vi "MNIST_Read_Dataset(as3D_refs).vi"(7 "MNIST Dataset Path":path=path "D:/DNN/data/DataSets/MNIST/train-images.idx3-ubyte", 8 "error in":errorcluster, 10 "Validation_Size":sgl=0.1) -> (0 "error out":errorcluster, 3 "Data(3D)_Refs":T1={"Train"={"Inputs Ref."=variant(refnum<data-value> refnum), "Outputs Ref."=refnum, "Dataset_Size"=0, "Dims_In"={"C"=0, "H"=0, "W"=0}, "Dims_Out"=0, "Labels"=[], "File Paths"=[]}, "Validation"={"Inputs Ref."=variant(refnum<data-value> refnum), "Outputs Ref."=refnum, "Dataset_Size"=0, "Dims_In"={"C"=0, "H"=0, "W"=0}, "Dims_Out"=0, "Labels"=[], "File Paths"=[]}, "Test"={"Inputs Ref."=variant(refnum<data-value> refnum), "Outputs Ref."=refnum, "Dataset_Size"=0, "Dims_In"={"C"=0, "H"=0, "W"=0}, "Dims_Out"=0, "Labels"=[], "File Paths"=[]}})   [LabVIEW 2024]
doc: "References to the dataset (Training, Validation and Testing)"
uses:
  <vilib>/Ngene/Deep Learning Toolkit/Toolkit/NN_Data/API/DataSet/DataSet_Types/NN_DataSets_All(In3D_Out1D).ctl
  <vilib>/Ngene/Deep Learning Toolkit/Toolkit/NN_Data/API/DataSet/DataSet_Types/NN_DataSet(In3D_Out1D).ctl
  <vilib>/Ngene/Deep Learning Toolkit/Toolkit/NN_Data/Controls/DataRef_Types/2D/NN_Data_ref(2D_SGL).ctl
  <vilib>/Ngene/Deep Learning Toolkit/Toolkit/NN_Data/API/NN_Dims(C,H,W).ctl
  <vilib>/Ngene/Deep Learning Toolkit/Toolkit/NN_Data/subVIs/Dataset_Split/NN_DataSet_Split(In3D_Out1D).vi
  <vilib>/Ngene/Deep Learning Toolkit/Toolkit/Deep_Learning_Toolkit_by_Ngene.lvlib
panel:
  # "Instructions:\n1. Download MNIST dataset from http://yann.lecun.com/exdb/mnist/  (4 files with .gz extension)\n2. Extract all 4 files in one folder\n3.  Provide corresponding path to 4 path controls below"
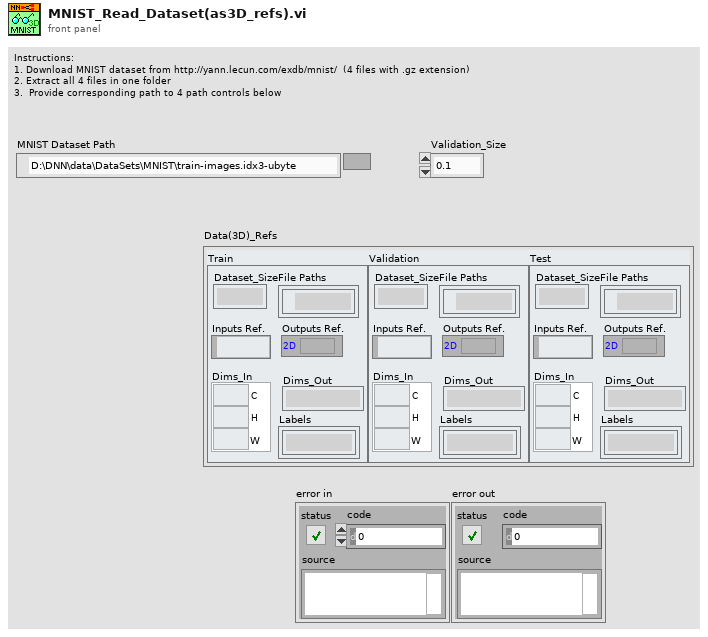
[diagram p1: front panel]
types:
  T1 = typedef "Deep_Learning_Toolkit_by_Ngene.lvlib/NN_DataSets_All(In3D_Out1D).ctl" = cluster{"Train":T2, "Validation":T2, "Test":T2}
  T2 = typedef "Deep_Learning_Toolkit_by_Ngene.lvlib/NN_DataSet(In3D_Out1D).ctl" = cluster{"Inputs Ref.":variant, "Outputs Ref.":T3, "Dataset_Size":i32, "Dims_In":T4, "Dims_Out":i32, "Labels":string[], "File Paths":path[]}
  T3 = typedef "Deep_Learning_Toolkit_by_Ngene.lvlib/NN_Data_ref(2D_SGL).ctl" = refnum<data-value>
  T4 = typedef "Deep_Learning_Toolkit_by_Ngene.lvlib/NN_Dims(C,H,W).ctl" = cluster{"C":i32, "H":i32, "W":i32}
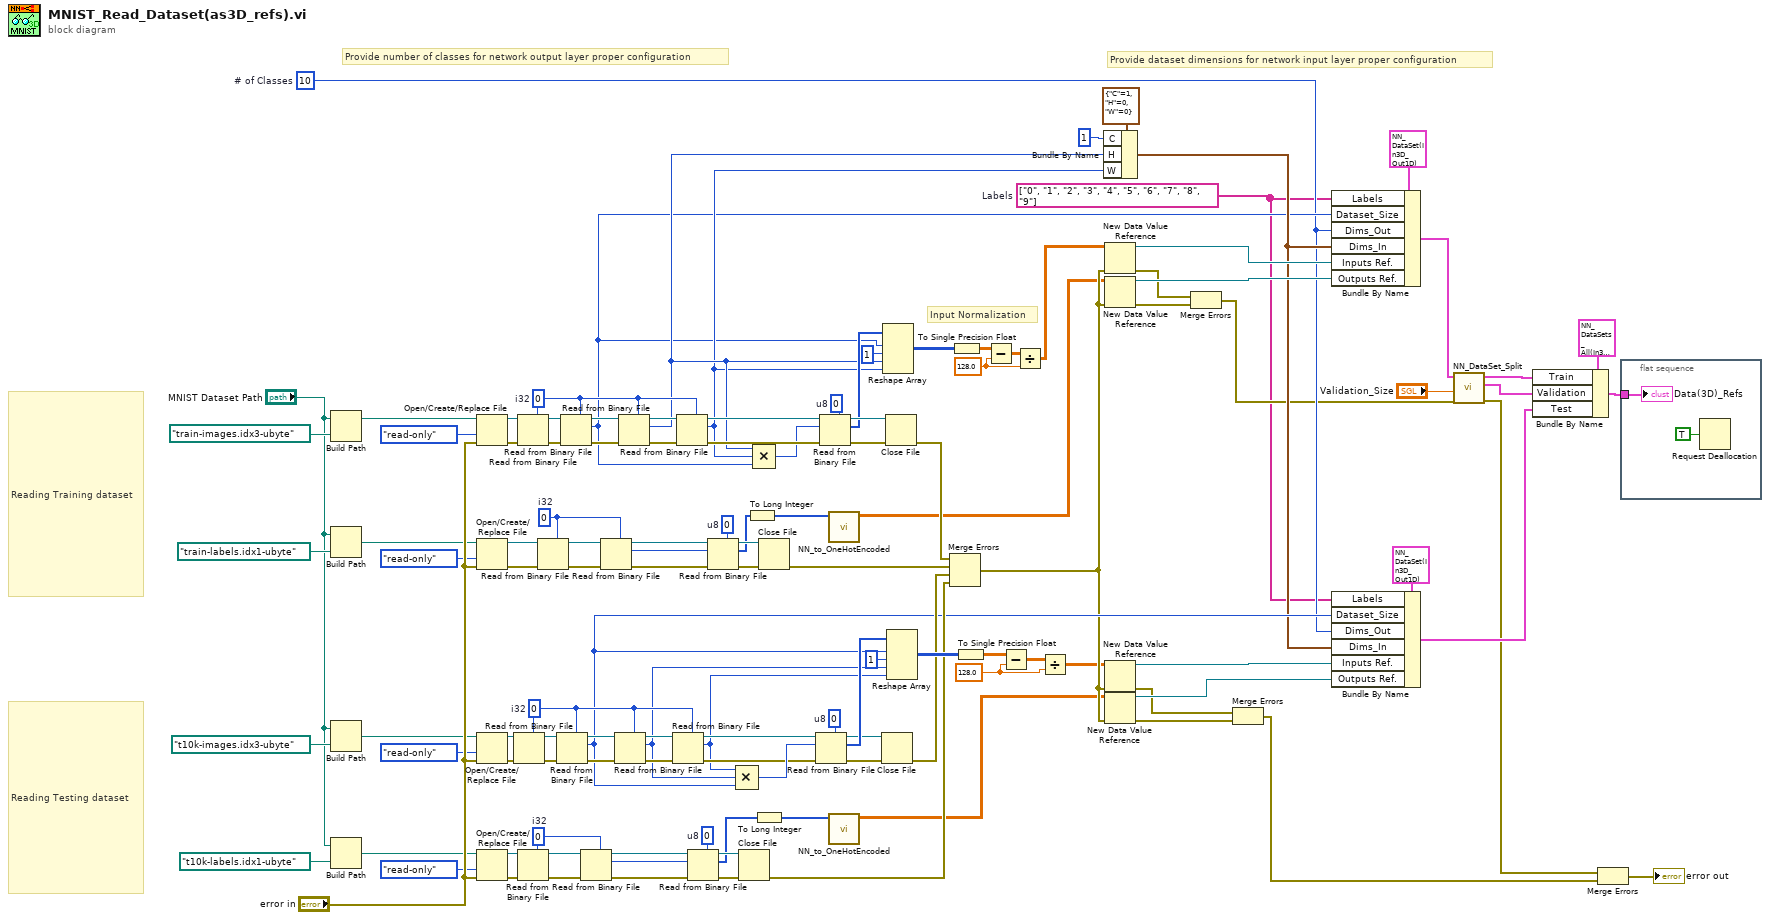
[diagram p0: block diagram]
diagram:
  w5 = string[] ["0", "1", "2", "3", "4", "5", "6", "7", "8", "9"]  # Labels
  w22 = sgl 128.0 ("y")
  w24 = sgl 128.0 ("y")
  w12 = 10  # # of Classes
  w94 = u8 0  # u8
  w93 = u8 0  # u8
  w85 = 0  # i32
  w74 = 0  # i32
  w98 = u8 0  # u8
  w99 = u8 0  # u8
  w107 = 0  # i32
  w118 = 0  # i32
  # "Provide dataset dimensions for network input layer proper configuration"
  # "Provide number of classes for network output layer proper configuration"
  # "Reading Testing dataset"
  # "Reading Training dataset"
  # "Input Normalization"
  n1 = Build Path(base path="MNIST Dataset Path", name or relative path=path "train-images.idx3-ubyte" ("Train_Label_Path")) -> (appended path=w21:path)
  n2 = Build Path(base path="MNIST Dataset Path", name or relative path=path "train-labels.idx1-ubyte" ("Train_Label_Path")) -> (appended path=w20:path)
  n3 = Build Path(base path="MNIST Dataset Path", name or relative path=path "t10k-images.idx3-ubyte" ("Test_Image_Path")) -> (appended path=w17:path)
  n4 = Build Path(base path="MNIST Dataset Path", name or relative path=path "t10k-labels.idx1-ubyte" ("Test_Label_Path")) -> (appended path=w14:path)
  n5 = Open/Create/Replace File(file path (use dialog)=w21, error in="error in", access (0:read/write)=enum16{"read/write", "read-only", "write-only"}."read-only") -> (refnum out=w122:refnum<file>, error out=w116:errorcluster)  [unwired: 3 in, 1 out]
  n6 = Open/Create/Replace File(file path (use dialog)=w20, error in="error in", access (0:read/write)=enum16{"read/write", "read-only", "write-only"}."read-only") -> (refnum out=w105:refnum<file>, error out=w108:errorcluster)  [unwired: 3 in, 1 out]
  n7 = Open/Create/Replace File(file path (use dialog)=w17, error in="error in", access (0:read/write)=enum16{"read/write", "read-only", "write-only"}."read-only") -> (refnum out=w70:refnum<file>, error out=w76:errorcluster)  [unwired: 3 in, 1 out]
  n8 = Open/Create/Replace File(file path (use dialog)=w14, error in="error in", access (0:read/write)=enum16{"read/write", "read-only", "write-only"}."read-only") -> (refnum out=w87:refnum<file>, error out=w84:errorcluster)  [unwired: 3 in, 1 out]
  n9 = Read from Binary File(5:w74, 8:w76, 11:w70) -> (0:w77:errorcluster, 3:w71:refnum<file>)  [unwired: 3 in, 2 out]
  n10 = Read from Binary File(5:w118, 8:w116, 11:w122) -> (0:w115:errorcluster, 3:w121:refnum<file>)  [unwired: 3 in, 2 out]
  n11 = Read from Binary File(5:w85, 8:w84, 11:w87) -> (0:w83:errorcluster, 3:w86:refnum<file>)  [unwired: 3 in, 2 out]
  n12 = Read from Binary File(5:w107, 8:w108, 11:w105) -> (0:w109:errorcluster, 3:w106:refnum<file>)  [unwired: 3 in, 2 out]
  n13 = Read from Binary File(5:w74, 8:w77, 11:w71) -> (0:w78:errorcluster, 2:w49:i32, 3:w73:refnum<file>)  [unwired: 3 in, 1 out]
  n14 = Read from Binary File(5:w118, 8:w115, 11:w121) -> (0:w114:errorcluster, 2:w26:i32, 3:w119:refnum<file>)  [unwired: 3 in, 1 out]
  n15 = Read from Binary File(5:w85, 8:w83, 11:w86) -> (0:w89:errorcluster, 2:w43:i32, 3:w88:refnum<file>)  [unwired: 3 in, 1 out]
  n16 = Read from Binary File(5:w107, 8:w109, 11:w106) -> (0:w103:errorcluster, 2:w44:i32, 3:w104:refnum<file>)  [unwired: 3 in, 1 out]
  n17 = Read from Binary File(5:w74, 8:w78, 11:w73) -> (0:w79:errorcluster, 2:w35:i32, 3:w72:refnum<file>)  [unwired: 3 in, 1 out]
  n18 = Read from Binary File(5:w118, 8:w114, 11:w119) -> (0:w113:errorcluster, 2:w30:i32, 3:w120:refnum<file>)  [unwired: 3 in, 1 out]
  n19 = Read from Binary File(5:w74, 8:w79, 11:w72) -> (0:w80:errorcluster, 2:w34:i32, 3:w75:refnum<file>)  [unwired: 3 in, 1 out]
  n20 = Read from Binary File(5:w118, 8:w113, 11:w120) -> (0:w112:errorcluster, 2:w29:i32, 3:w117:refnum<file>)  [unwired: 3 in, 1 out]
  n21 = Read from Binary File(5:w94, 8:w89, 10:w43, 11:w88) -> (0:w91:errorcluster, 2:w42:u8[], 3:w90:refnum<file>)  [unwired: 2 in, 1 out]
  n22 = Read from Binary File(5:w98, 8:w103, 10:w44, 11:w104) -> (0:w101:errorcluster, 2:w96:u8[], 3:w102:refnum<file>)  [unwired: 2 in, 1 out]
  n23 = Compound Arithmetic op=MULTIPLY(w34, w35, w49) -> (w82:i32)
  n24 = Close File(refnum=w90, error in=w91) -> (error out=w57:errorcluster)  [unwired: 1 out]
  n25 = To Long Integer(number=w96) -> (32bit integer=w2:i32[])
  n26 = Compound Arithmetic op=MULTIPLY(w30, w29, w26) -> (w110:i32)
  n27 = To Long Integer(number=w42) -> (32bit integer=w4:i32[])
  n28 = Close File(refnum=w102, error in=w101) -> (error out=w59:errorcluster)  [unwired: 1 out]
  n29 = Read from Binary File(5:w93, 8:w80, 10:w82, 11:w75) -> (0:w81:errorcluster, 2:w92:u8[], 3:w69:refnum<file>)  [unwired: 2 in, 1 out]
  n30 = Read from Binary File(5:w99, 8:w112, 10:w110, 11:w117) -> (0:w111:errorcluster, 2:w100:u8[], 3:w123:refnum<file>)  [unwired: 2 in, 1 out]
  n31 = call <vilib>:"NN_to_OneHotEncoded.vi"("Label_Idx"=w2) -> ("Prediction"=w1:sgl[][])  [unwired: 10 in]
  n32 = call <vilib>:"NN_to_OneHotEncoded.vi"("Label_Idx"=w4) -> ("Prediction"=w3:sgl[][])  [unwired: 10 in]
  n33 = Close File(refnum=w69, error in=w81) -> (error out=w58:errorcluster)  [unwired: 1 out]
  n34 = Reshape Array(w100, w26, 1 ("dimension size"), w30, w29) -> (w97:u8[][][][])
  n35 = Close File(refnum=w123, error in=w111) -> (error out=w60:errorcluster)  [unwired: 1 out]
  n36 = Reshape Array(w92, w49, 1 ("dimension size"), w35, w34) -> (w95:u8[][][][])
  n37 = Merge Errors(w60, w59, w58, w57) -> (w41:errorcluster)
  n38 = To Single Precision Float(number=w97) -> (single precision float=w61:sgl[][][][])
  n39 = To Single Precision Float(number=w95) -> (single precision float=w62:sgl[][][][])
  n40 = Subtract(x=w61, y=w24) -> (x-y=w36:sgl[][][][])
  n41 = Subtract(x=w62, y=w22) -> (x-y=w37:sgl[][][][])
  n42 = Divide(x=w36, y=w24) -> (x/y=w25:sgl[][][][])
  n43 = Divide(x=w37, y=w22) -> (x/y=w23:sgl[][][][])
  n44 = Bundle By Name(cluster=T4 {"C"=1, "H"=0, "W"=0} ("Dims"), "C"=1 ("Chs"), "H"=w30, "W"=w29) -> (w28:T4)
  n45 = New Data Value Reference(data value=w25, error in=w41) -> (data value reference=w67:refnum<data-value>, error out=w55:errorcluster)
  n46 = New Data Value Reference(data value=w1, error in=w41) -> (data value reference=w66:refnum<data-value>, error out=w56:errorcluster)
  n47 = New Data Value Reference(data value=w23, error in=w41) -> (data value reference=w64:refnum<data-value>, error out=w54:errorcluster)
  n48 = New Data Value Reference(data value=w3, error in=w41) -> (data value reference=w65:refnum<data-value>, error out=w53:errorcluster)
  n49 = Merge Errors(w55, w56) -> (w11:errorcluster)
  n50 = Merge Errors(w54, w53) -> (w52:errorcluster)
  n51 = Bundle By Name(cluster=T2 {"Inputs Ref."=variant(refnum<data-value> refnum), "Outputs Ref."=refnum, "Dataset_Size"=0, "Dims_In"={"C"=0, "H"=0, "W"=0}, "Dims_Out"=0, "Labels"=[], "File Paths"=[]} ("Test_Data"), "Labels"=w5, "Dataset_Size"=w26, "Dims_Out"=w12, "Dims_In"=w28, "Inputs Ref."=w67, "Outputs Ref."=w66) -> (w9:T2)
  n52 = Bundle By Name(cluster=T2 {"Inputs Ref."=variant(refnum<data-value> refnum), "Outputs Ref."=refnum, "Dataset_Size"=0, "Dims_In"={"C"=0, "H"=0, "W"=0}, "Dims_Out"=0, "Labels"=[], "File Paths"=[]} ("Test_Data"), "Labels"=w5, "Dataset_Size"=w49, "Dims_Out"=w12, "Dims_In"=w28, "Inputs Ref."=w64, "Outputs Ref."=w65) -> (w40:T2)
  n53 = call-poly <vilib>:"NN_DataSet_Split.vi"("error in(no error)"=w11, "Split Size"="Validation_Size", "Dataset In"=w9) -> ("error out"=w6:errorcluster, "Dataset Out 2"=w7:T2, "Dataset Out 1"=w8:T2)  [unwired: 6 in]
  n54 = Bundle By Name(cluster=T1 {"Train"={"Inputs Ref."=variant(refnum<data-value> refnum), "Outputs Ref."=refnum, "Dataset_Size"=0, "Dims_In"={"C"=0, "H"=0, "W"=0}, "Dims_Out"=0, "Labels"=[], "File Paths"=[]}, "Validation"={"Inputs Ref."=variant(refnum<data-value> refnum), "Outputs Ref."=refnum, "Dataset_Size"=0, "Dims_In"={"C"=0, "H"=0, "W"=0}, "Dims_Out"=0, "Labels"=[], "File Paths"=[]}, "Test"={"Inputs Ref."=variant(refnum<data-value> refnum), "Outputs Ref."=refnum, "Dataset_Size"=0, "Dims_In"={"C"=0, "H"=0, "W"=0}, "Dims_Out"=0, "Labels"=[], "File Paths"=[]}} ("Data_Refs"), "Train"=w8, "Validation"=w7, "Test"=w40) -> (w39:T1)
  n55 = Merge Errors(w6, w52) -> (→"error out":errorcluster)
  n56 = flat-sequence {
    tunnel: w39 -> [w125]
    frame #0 {
      n57 = Request Deallocation(TRUE ("flag")) -> ()
      "Data(3D)_Refs" <- w125
    }
  }
